vi "Round4thDecimal.vi"(11 "Double Float":dbl) -> (3 "Rounded Value":dbl)   [LabVIEW 2014]
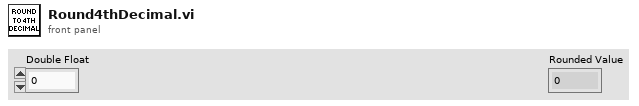
[diagram p1: front panel]
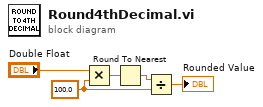
[diagram p0: block diagram]
diagram:
  w3 = 100.0 ("y")
  n1 = Multiply(x="Double Float", y=w3) -> (x*y=w5:dbl)
  n2 = Round To Nearest(number=w5) -> (nearest integer value=w4:dbl)
  n3 = Divide(x=w4, y=w3) -> (x/y=→"Rounded Value":dbl)
